vi "slowinit.vi"(8 "UTC format":bool=TRUE, 9 "XOFF Character":u8=19 format="%.0x", 10 "XON Character":u8=17 format="%.0x", 11 "VISA resource name":refnum<visa-resource-name>="COM5") -> (0 "error IO":errorcluster, 3 "VISA resource name out":refnum<visa-resource-name>, 7 "Slow Cluster":T1={"Number of Slow Parameters"=0, "UTC format?"=TRUE, "Sensor Upper bounds"=[85, 1000000, 8000, 8000, 8000, 14000, 99, 33000], "Sensor Lower bounds"=[-40, 0, -8000, -8000, -8000, -14000, 0, -33000], "datanames"=[], "Descriptions"=[]})   [LabVIEW 2012]
uses:
  <vilib>/Instr/_visa.llb/VISA Configure Serial Port (Instr).vi
panel:
  in  "Slow Cluster 2":T1={"Number of Slow Parameters"=0, "UTC format?"=TRUE, "Sensor Upper bounds"=[85, 1000000, 8000, 8000, 8000, 14000, 99, 33000], "Sensor Lower bounds"=[-40, 0, -8000, -8000, -8000, -14000, 0, -33000], "datanames"=[], "Descriptions"=[]}
  out "Datanames":string[](array[string])
  out "Description":string[](array[string])
  out "Up bound":i32[](array[numeric])
  out "Low bound":i32[](array[numeric])
  out "Stopped":bool
  out "array of datanames":string[](array[string])
  out "array of datanames 2":string[](array[string])
  out "Arduino needs to be reinitialized":bool
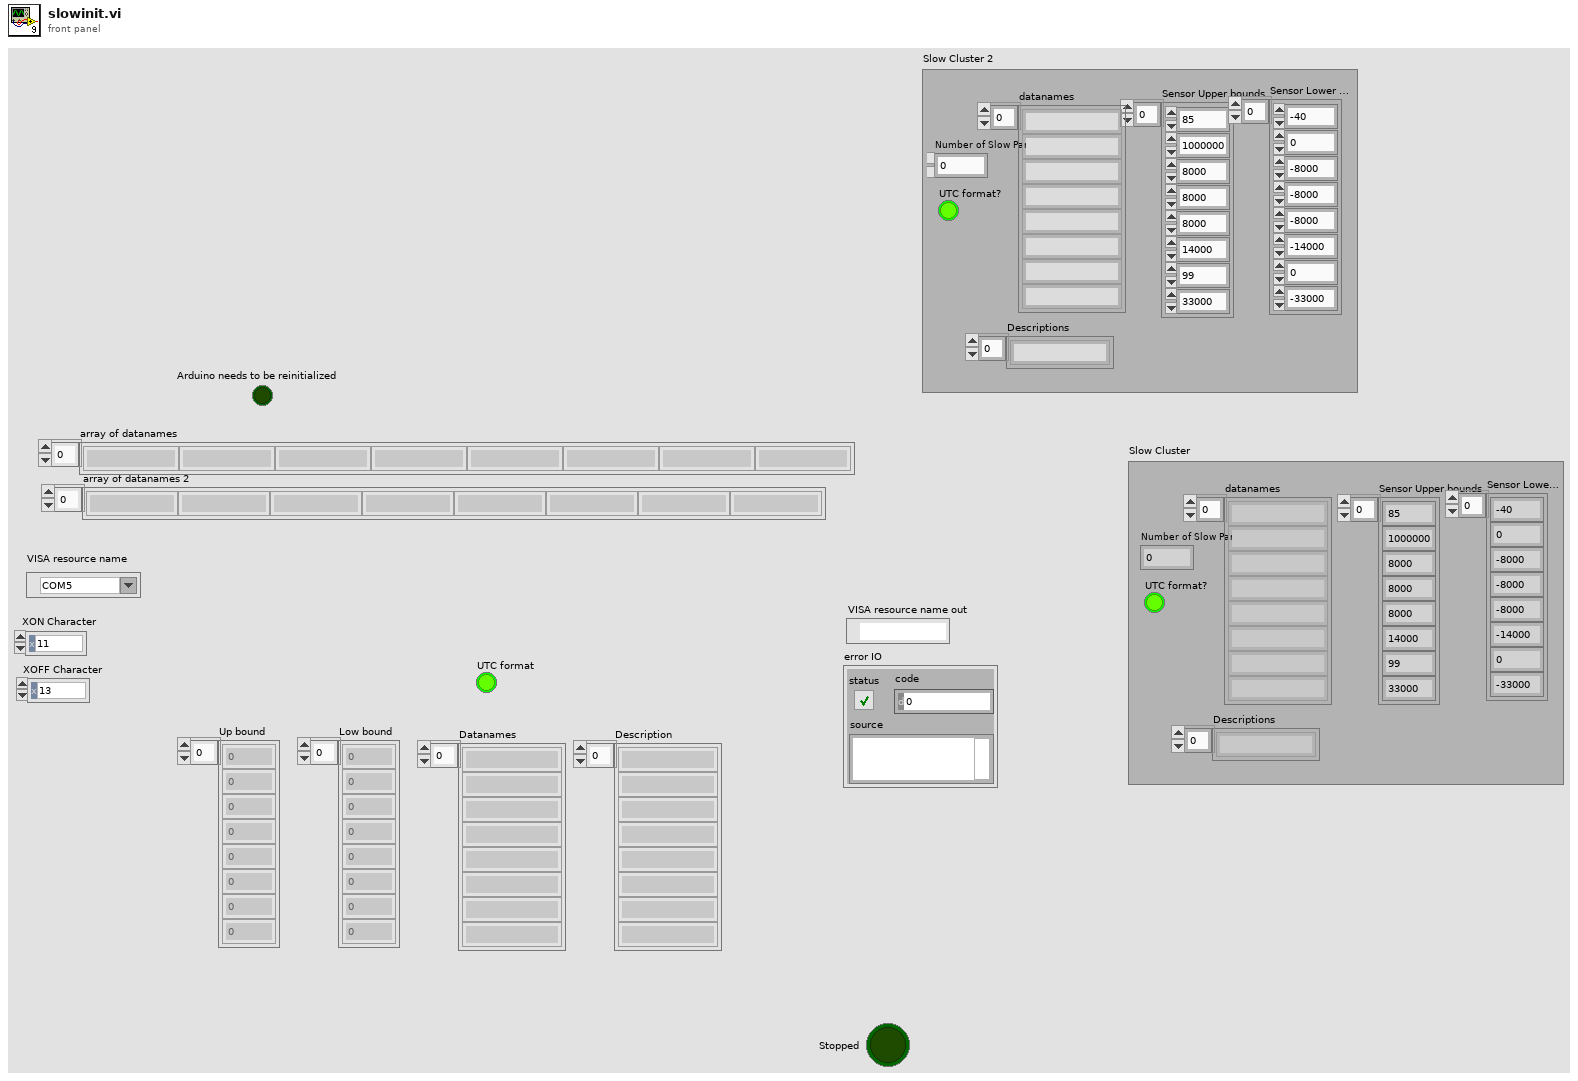
[diagram p1: front panel]
types:
  T1 = cluster{"Number of Slow Parameters":i32, "UTC format?":bool, "Sensor Upper bounds":i32[], "Sensor Lower bounds":i32[], "datanames":string[], "Descriptions":string[]}
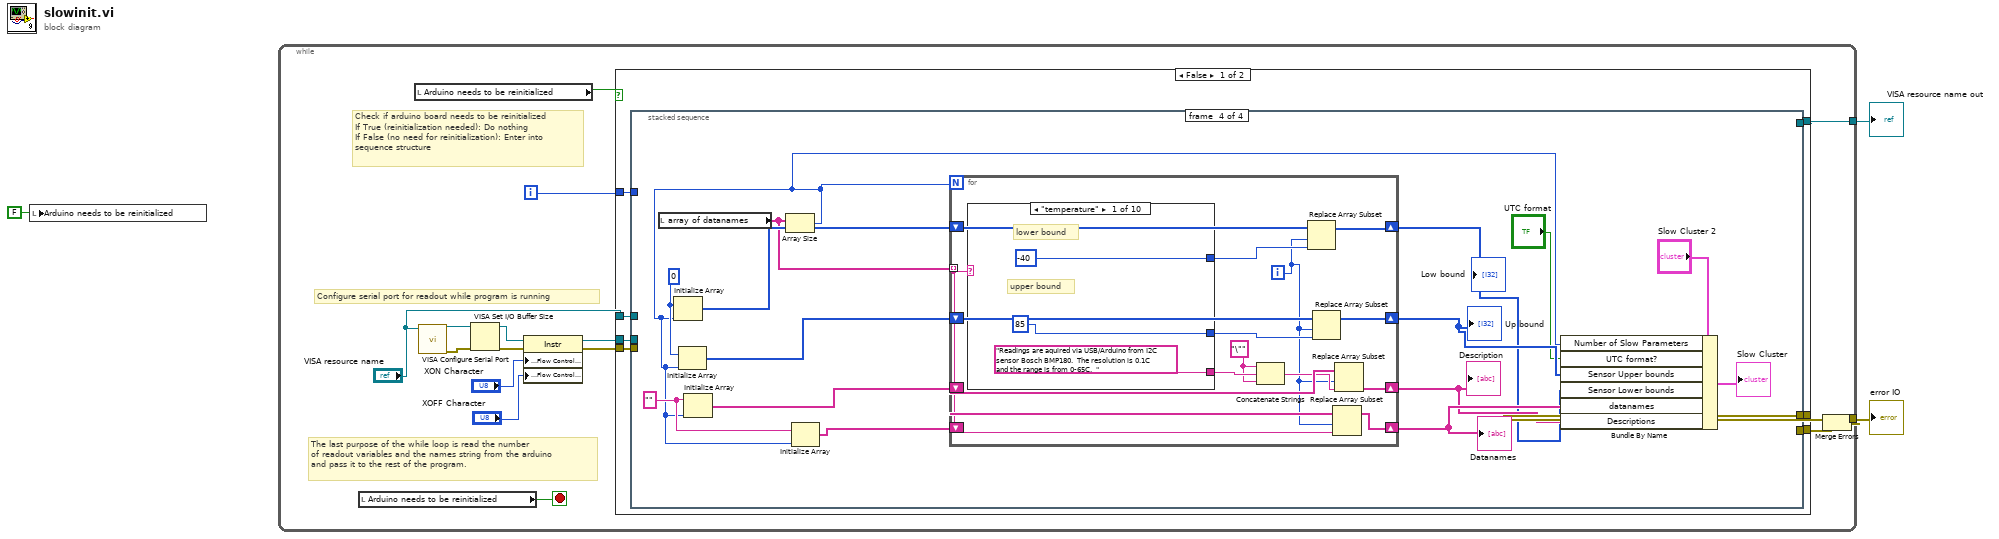
[diagram p0: block diagram]
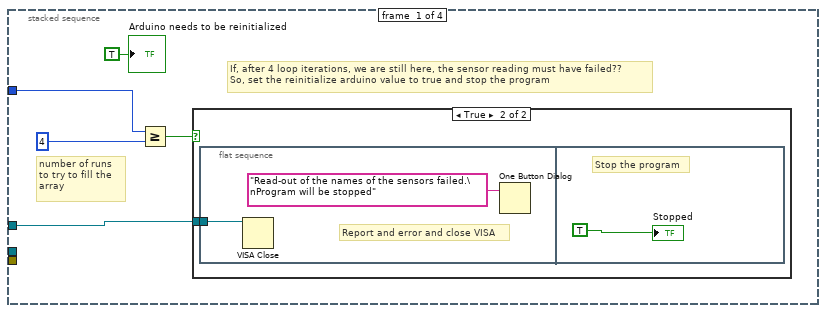
[diagram p2: hidden frame]
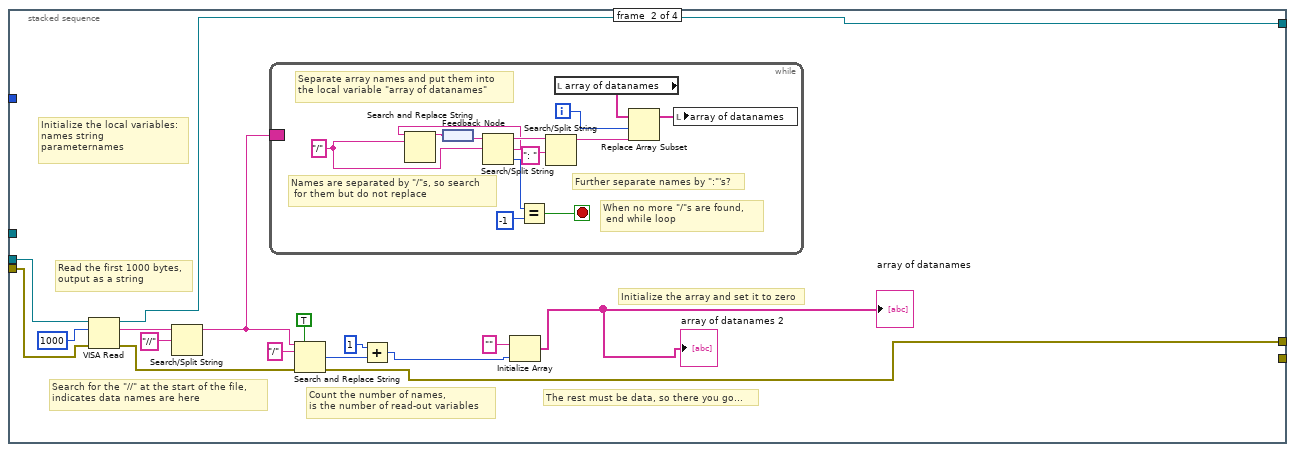
[diagram p4: hidden frame]
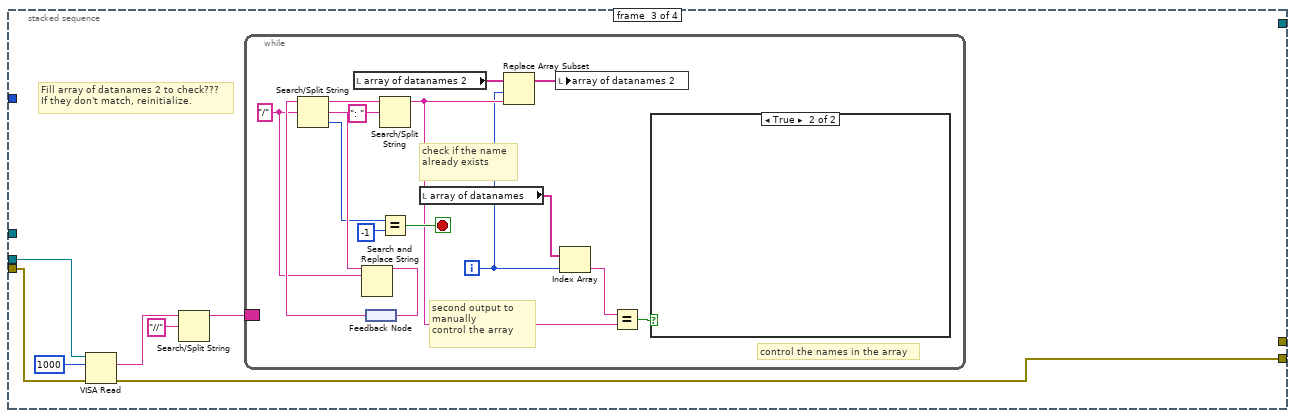
[diagram p5: hidden frame]
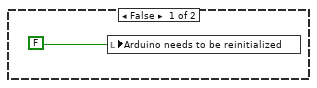
[diagram p6: hidden frame]
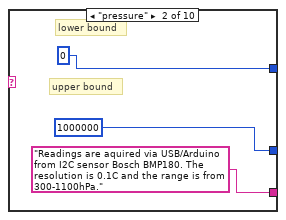
[diagram p7: hidden frame]
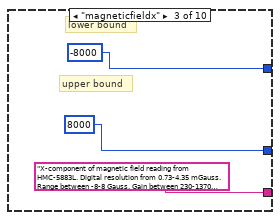
[diagram p8: hidden frame]
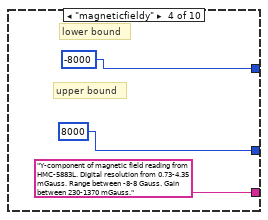
[diagram p9: hidden frame]
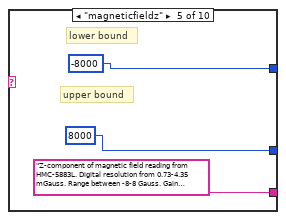
[diagram p10: hidden frame]
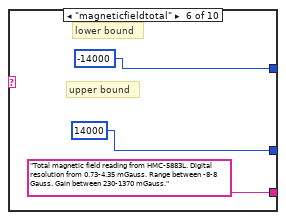
[diagram p11: hidden frame]
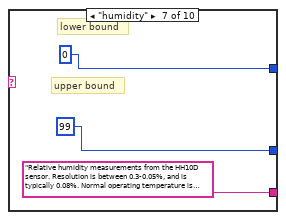
[diagram p12: hidden frame]
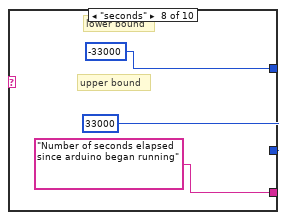
[diagram p13: hidden frame]
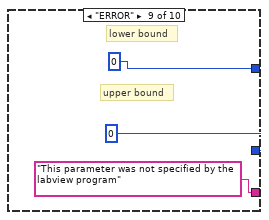
[diagram p14: hidden frame]
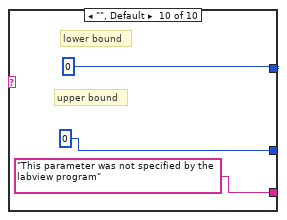
[diagram p15: hidden frame]
diagram:
  n1 = local write "Arduino needs to be reinitialized"(FALSE ("Arduino needs to be reinitialized")) -> ()
  n2 = while {
    tunnel: [w13] -> w3
    tunnel: [w12] -> w2
    i -> [w10]
    stop <- w8 stop-if-true
    # "The last purpose of the while loop is read the number \nof readout variables and the names string from the arduino\nand pass it to the rest of the program."
    # "Check if arduino board needs to be reinitialized\nIf True (reinitialization needed): Do nothing\nIf False (no need for reinitialization): Enter into \nsequence structure"
    # "Configure serial port for readout while program is running"
    n3 = local read "Arduino needs to be reinitialized"() -> (w8:bool)
    n4 = local read "Arduino needs to be reinitialized"() -> (w7:bool)
    n5 = call-poly "VISA Configure Serial Port"("VISA resource name"="VISA resource name") -> ("VISA resource name out"=w15:refnum<visa-resource-name>, "error out"=w14:errorcluster)  [unwired: 9 in, 4 out]
    n6 = VISA Set I/O Buffer Size(VISA resource name=w15, error in (no error)=w14) -> (VISA resource name out=w19:refnum<visa-resource-name>, error out=w18:errorcluster)  [unwired: 2 in]
    n7 = property class="Instr"(reference=w19, error in=w18, "Serial Settings:Flow Control XON Character"="XON Character", "Serial Settings:Flow Control XOFF Character"="XOFF Character") -> (reference out=w11:refnum<visa-resource-name>, error out=w6:errorcluster)
    n8 = case shown="False" w7 {
      tunnel: [w26 w149] -> w13
      tunnel: w11 -> [w25 w149]
      tunnel: w10 -> [w24 _]
      tunnel: "VISA resource name" -> [w23 _]
      tunnel: w6 -> [w22 _]
      tunnel: [w21 _] -> w5
      tunnel: [w20 _] -> w4
      frame False {
        n9 = stacked-sequence {
          tunnel: [_ w48 _ _] -> w26
          tunnel: w25 -> [_ w51 w68 _]
          tunnel: w24 -> [w31 _ _ _]
          tunnel: w23 -> [w28 _ _ _]
          tunnel: w22 -> [_ w49 w66 _]
          tunnel: [_ w38 _ _] -> w21
          tunnel: [_ _ w65 _] -> w20
          frame #0 {
            # "If, after 4 loop iterations, we are still here, the sensor reading must have failed??  \nSo, set the reinitialize arduino value to true and stop the program"
            # "number of runs to try to fill the array"
            n10 = Greater Or Equal?(x=w31, y=4) -> (x >= y?=w29:bool)
            n11 = case shown="True" w29 {
              tunnel: w28 -> [_ w32]
              frame False {
              }
              frame True {
                n12 = flat-sequence {
                  tunnel: w32 -> [w33]
                  frame #0 {
                    # "Report and error and close VISA"
                    n13 = VISA Close(VISA resource name=w33) -> ()  [unwired: 1 in, 1 out]
                    n14 = One Button Dialog(message="Read-out of the names of the sensors failed.\nProgram will be stopped") -> ()  [unwired: 1 in, 1 out]
                  }
                  frame #1 {
                    # "Stop the program"
                    "Stopped" <- TRUE ("stop? (T)")
                  }
                }
              }
            }
            "Arduino needs to be reinitialized" <- TRUE ("Arduino needs to be reinitialized")
          }
          frame #1 {
            # "The rest must be data, so there you go..."
            # "Count the number of names, \nis the number of read-out variables"
            # "Search for the \"//\" at the start of the file, \nindicates data names are here"
            # "Initialize the local variables: \nnames string\nparameternames"
            # "Read the first 1000 bytes, \noutput as a string"
            # "Initialize the array and set it to zero"
            n15 = VISA Read(VISA resource name=w51, byte count=u32 1000, error in (no error)=w49) -> (VISA resource name out=w48:refnum<visa-resource-name>, read buffer=w47:string, error out=w39:errorcluster)  [unwired: 1 out]
            n16 = Search/Split String(string=w47, search string/char (-)="//") -> (substring before match=w43:string)  [unwired: 1 in, 2 out]
            n17 = while {
              border: w43 -> [_]
              i -> [w52]
              stop <- w61 stop-if-true
              w57 = "/" ("search string/char (-)")
              # "Further separate names by \":\"'s?"
              # "When no more \"/\"s are found,\n end while loop"
              # "Names are separated by \"/\"s, so search\n for them but do not replace"
              # "Separate array names and put them into \nthe local variable \"array of datanames\""
              n18 = feedback #1() -> (w59:string)
              n19 = Search/Split String(string=w59, search string/char (-)=w57) -> (substring before match=w55:string, match + rest of string=w54:string, offset of match=w56:i32)  [unwired: 1 in]
              n20 = Search and Replace String(input string=w54, search string=w57) -> (result string=w58:string)  [unwired: 6 in, 3 out]
              n21 = feedback-in #1(w58) -> ()
              n22 = Equal?(x=w56, y=-1) -> (x = y?=w61:bool)
              n23 = Search/Split String(string=w55, search string/char (-)=": " ("format string")) -> (substring before match=w53:string)  [unwired: 1 in, 2 out]
              n24 = local read "array of datanames"() -> (w63:string[])
              n25 = Replace Array Subset(array=w63, new element=w53, index=w52) -> (w62:string[])
              n26 = local write "array of datanames"(w62) -> ()
            }
            n27 = Search and Replace String(replace all?=TRUE ("replace all? (F)"), input string=w43, search string="/", error in=w39) -> (number of replacements=w44:i32, error out=w38:errorcluster)  [unwired: 4 in, 2 out]
            n28 = Add(x=1, y=w44) -> (x+y=w36:i32)
            n29 = Initialize Array("", w36) -> (→"array of datanames" →"array of datanames 2":string[])
          }
          frame #2 {
            # "Fill array of datanames 2 to check???\nIf they don't match, reinitialize."
            n30 = VISA Read(VISA resource name=w68, byte count=u32 1000, error in (no error)=w66) -> (read buffer=w71:string, error out=w65:errorcluster)  [unwired: 2 out]
            n31 = Search/Split String(string=w71, search string/char (-)="//") -> (substring before match=w67:string)  [unwired: 1 in, 2 out]
            n32 = while {
              border: w67 -> [_]
              i -> [w72]
              stop <- w83 stop-if-true
              w78 = "/" ("search string/char (-)")
              # "second output to manually\ncontrol the array"
              # "check if the name already exists"
              # "control the names in the array"
              n33 = local read "array of datanames 2"() -> (w85:string[])
              n34 = feedback #2() -> (w81:string)
              n35 = Search/Split String(string=w81, search string/char (-)=w78) -> (substring before match=w86:string, match + rest of string=w80:string, offset of match=w77:i32)  [unwired: 1 in]
              n36 = Search and Replace String(input string=w80, search string=w78) -> (result string=w79:string)  [unwired: 6 in, 3 out]
              n37 = feedback-in #2(w79) -> ()
              n38 = Search/Split String(string=w86, search string/char (-)=": " ("format string")) -> (substring before match=w74:string)  [unwired: 1 in, 2 out]
              n39 = Equal?(x=w77, y=-1) -> (x = y?=w83:bool)
              n40 = local read "array of datanames"() -> (w75:string[])
              n41 = Replace Array Subset(array=w85, new element=w74, index=w72) -> (w84:string[])
              n42 = local write "array of datanames 2"(w84) -> ()
              n43 = Index Array(array=w75, index=w72) -> (element=w76:string)
              n44 = Equal?(x=w76, y=w74) -> (x = y?=w73:bool)
              n45 = case shown="True" w73 {
                frame False {
                  n46 = local write "Arduino needs to be reinitialized"(FALSE ("reinitialize arduino read boolean")) -> ()
                }
                frame True {
                }
              }
            }
          }
          frame #3 {
            w97 = ""
            w103 = 0 ("element")
            n47 = local read "array of datanames"() -> (w98:string[])
            n48 = Array Size(array=w98) -> (size(s)=w92:i32)
            n49 = Initialize Array(w103, w92) -> (w102:i32[])
            n50 = Initialize Array(w103, w92) -> (w101:i32[])
            n51 = Initialize Array(w97, w92) -> (w100:string[])
            n52 = Initialize Array(w97, w92) -> (w99:string[])
            n53 = for {
              N: w92 -> [_]
              tunnel: w98 -> [w104] mode=indexing
              shift-right: [w113] -> w94
              shift-left: w101 -> [w117]
              shift-right: [w114] -> w93
              shift-left: w102 -> [w118]
              shift-right: [w111] -> w95
              shift-left: w100 -> [w112]
              shift-right: [w105] -> w96
              shift-left: w99 -> [w107]
              i -> [w106]
              w109 = "\"" ("string")
              n54 = case shown="\"temperature\"" w104 {
                tunnel: [85 1000000 8000 8000 8000 14000 99 33000 0 0] -> w115
                tunnel: [-40 0 -8000 -8000 -8000 -14000 0 -33000 0 0] -> w116
                tunnel: ["Readings are aquired via USB/Arduino from I2C sensor Bosch BMP180.  The resolution is 0.1C and the range is from 0-65C.  " ("XML Tag") "Readings are aquired via USB/Arduino from I2C sensor Bosch BMP180. The resolution is 0.1C and the range is from 300-1100hPa." "X-component of magnetic field reading from HMC-5883L. Digital resolution from 0.73-4.35 mGauss. Range between -8-8 Gauss. Gain between 230-1370 mGauss. " "Y-component of magnetic field reading from HMC-5883L. Digital resolution from 0.73-4.35 mGauss. Range between -8-8 Gauss. Gain between 230-1370 mGauss." "Z-component of magnetic field reading from HMC-5883L. Digital resolution from 0.73-4.35 mGauss. Range between -8-8 Gauss. Gain between 230-1370 mGauss." "Total magnetic field reading from HMC-5883L. Digital resolution from 0.73-4.35 mGauss. Range between -8-8 Gauss. Gain between 230-1370 mGauss." "Relative humidity measurements from the HH10D sensor. Resolution is between 0.3-0.05%, and is typically 0.08%. Normal operating temperature is 0-60C and the drift over time is 1% per year. " "Number of seconds elapsed since arduino began running" ("XML Tag") "This parameter was not specified by the labview program" ("XML Tag") "This parameter was not specified by the labview program" ("XML Tag")] -> w110
                frame "temperature" {
                  # "upper bound"
                  # "lower bound"
                }
                frame "pressure" {
                  # "upper bound"
                  # "lower bound"
                }
                frame "magneticfieldx" {
                  # "upper bound"
                  # "lower bound"
                }
                frame "magneticfieldy" {
                  # "upper bound"
                  # "lower bound"
                }
                frame "magneticfieldz" {
                  # "upper bound"
                  # "lower bound"
                }
                frame "magneticfieldtotal" {
                  # "upper bound"
                  # "lower bound"
                }
                frame "humidity" {
                  # "upper bound"
                  # "lower bound"
                }
                frame "seconds" {
                  # "upper bound"
                  # "lower bound"
                }
                frame "ERROR" {
                  # "upper bound"
                  # "lower bound"
                }
                frame "", Default {
                  # "upper bound"
                  # "lower bound"
                }
              }
              n55 = Concatenate Strings(w109, w110, w109) -> (w108:string)
              n56 = Replace Array Subset(array=w118, new element=w116, index=w106) -> (w114:i32[])
              n57 = Replace Array Subset(array=w117, new element=w115, index=w106) -> (w113:i32[])
              n58 = Replace Array Subset(array=w107, new element=w104, index=w106) -> (w105:string[])
              n59 = Replace Array Subset(array=w112, new element=w108, index=w106) -> (w111:string[])
            }
            "Low bound" <- w93
            "Up bound" <- w94
            "Description" <- w95
            "Datanames" <- w96
            n60 = Bundle By Name(cluster="Slow Cluster 2", "Number of Slow Parameters"=w92, "UTC format?"="UTC format", "Sensor Upper bounds"=w94, "Sensor Lower bounds"=w93, "datanames"=w96, "Descriptions"=w95) -> (→"Slow Cluster":T1)
          }
        }
      }
      frame True {
      }
    }
    n61 = Merge Errors(w5, w4) -> (w12:errorcluster)
  }
  "VISA resource name out" <- w3
  "error IO" <- w2
